vi "Velocity Change Command SubVi.vi"(2 "Acceleration":dbl, 3 "Velocity":dbl, 4 "error in":errorcluster, 5 "reference in":refnum<k24>) -> (0 "error out":errorcluster, 1 "reference out":refnum<k24>)   [LabVIEW 2017]
uses:
  Newport.XPS.CommandInterface
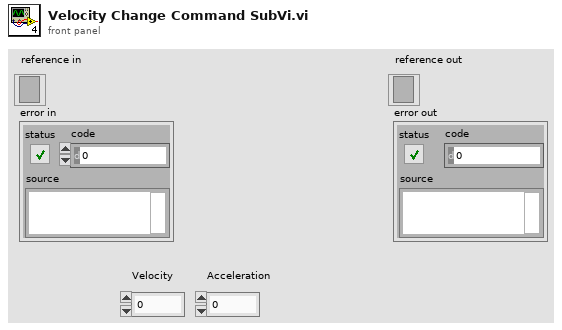
[diagram p1: front panel]
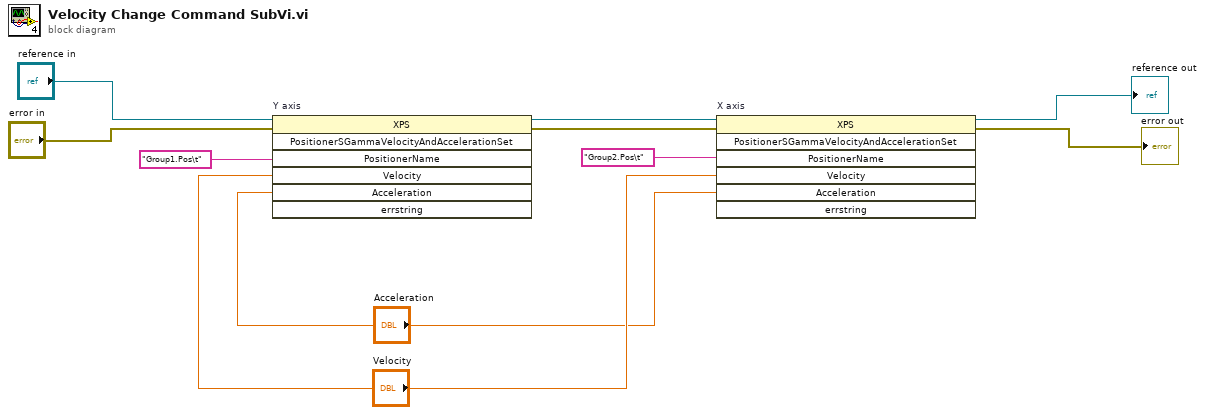
[diagram p0: block diagram]
diagram:
  n1 = invoke on="Y axis" class="XPS" method="PositionerSGammaVelocityAndAccelerationSet"(reference="reference in", error in="error in", "PositionerName"="Group1.Pos\t", "Velocity"="Velocity", "Acceleration"="Acceleration") -> (reference out=w8:refnum<k24>, error out=w7:errorcluster)  [unwired: 2 in, 5 out]
  n2 = invoke on="X axis" class="XPS" method="PositionerSGammaVelocityAndAccelerationSet"(reference=w8, error in=w7, "PositionerName"="Group2.Pos\t", "Velocity"="Velocity", "Acceleration"="Acceleration") -> (reference out=→"reference out":refnum<k24>, error out=→"error out":errorcluster)  [unwired: 2 in, 5 out]
